vi "List Headers.vi"(8 "error in (no error)":errorcluster, 11 "HTTP Client Base in":refnum<class "LabVIEW HTTP Client.lvclass">) -> (0 "error out":errorcluster, 2 "headers":string, 3 "HTTP Client Base out":refnum<class "LabVIEW HTTP Client.lvclass">)   [LabVIEW 2021, in "HTTP Client Abstract.lvlib" / "LabVIEW HTTP Client.lvclass"]
uses:
  LabVIEW HTTP Client.lvclass
  LabVIEW HTTP Client.lvclass/LabVIEW HTTP Client.ctl
  <vilib>/httpClient/LabVIEWHTTPClient.lvlib
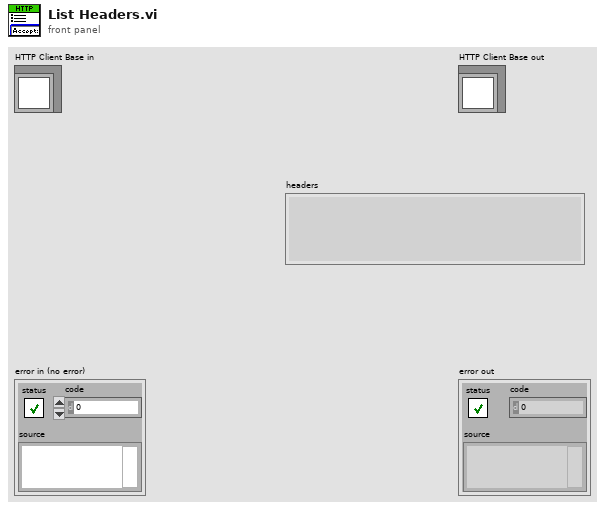
[diagram p1: front panel]
types:
  T1 = typedef "LabVIEWHTTPClient.lvlib/ClientHandle.ctl" = refnum<k1>
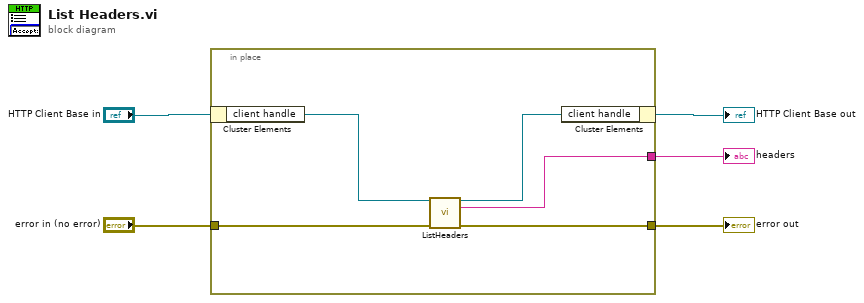
[diagram p0: block diagram]
diagram:
  n1 = in-place {
    in-place-border: "error in (no error)" -> [w10]
    in-place-border: [w9] -> w4
    in-place-border: [w6] -> w2
    n2 = in-place-cluster #1("HTTP Client Base in") -> ("client handle"=w8:T1)
    n3 = call <vilib>:"ListHeaders.vi"("client handle"=w8, "error in (no error)"=w10) -> ("client handle out"=w7:T1, "headers"=w6:string, "error out"=w9:errorcluster)  [unwired: 11 in]
    n4 = in-place-cluster #1("client handle"=w7) -> (→"HTTP Client Base out":refnum<class "LabVIEW HTTP Client.lvclass">)
  }
  "error out" <- w4
  "headers" <- w2
